vi "Main.vi"() -> ()   [LabVIEW 2018]
doc: "This Continuous Measurement sample project is based on the Queued Message Handler template.\n\nThe Event Handling Loop generates messages based on user interface actions.\n\nThe Message Handling Loop processes messages generated by the Event Handling Loop, or by other messages. There are also Acquisition and Logging message handling loop subVIs, and a chart updating loop."
uses:
  Controls/Acquired Data.ctl
  Controls/Time Remaining.ctl
  Controls/UI State.ctl
  Settings/Settings.ctl
  Acquisition/Hardware Configuration.ctl
  Logging/Logging Configuration.ctl
  <vilib>/addons/database/Connection.llb/Conn ObjectReference.ctl
  Support/Message Queue/Enqueue Message (Array).vi
  Support/Message Queue/Enqueue Message (Single).vi
  <vilib>/Utility/error.llb/Error Cluster From Error Code.vi
  <vilib>/ErrorRing/Error Ring.xnode
  Logging/Logging.lvlib
  Acquisition/Acquisition.lvlib
  Settings/Settings.lvlib
  support/User Event - Stop/User Event - Stop.lvlib
  support/Message Queue/Message Queue.lvlib
  <vilib>/addons/database/NI_Database_API.lvlib
  OSTEP_MySQLdBTools/MySQLTools.lvlib
  Settings/Settings Dialog.vi
panel:
  in  "UI State":T1
  out "Test In Progress":bool
  out "Time":T2 format="%<00:%M:%S>T"
  in  "Operator":u16(ring) items=["Select Operator"=0, "Wally Taylor"=2, "Max Ivanov"=3, "Scott Mowery"=4, "Robert Heitsenrether"=5, "Chris Haith"=6, "Chris McGrath"=7, "Kevin Harrison"=8, "Nathan Holcomb"=9, "Warren Krug"=10, "Winston Hensley"=11]
  in  "Location":u16(ring) items=["Chesapeake", "Silver Spring", "Gulf", "Seattle"]
  out "StatusBox":string
  out "Data":dbl(graph)
  in  "Range Data":T3={"offset"=99.0, "time"=""} {"offset" format="%.3g"}
  out "User Event - Stop":refnum<user-event>
  in  "Settings":bool
  in  "Start":bool
  in  "Stop":bool
  out "Status Bar":string
  in  "Exit":bool
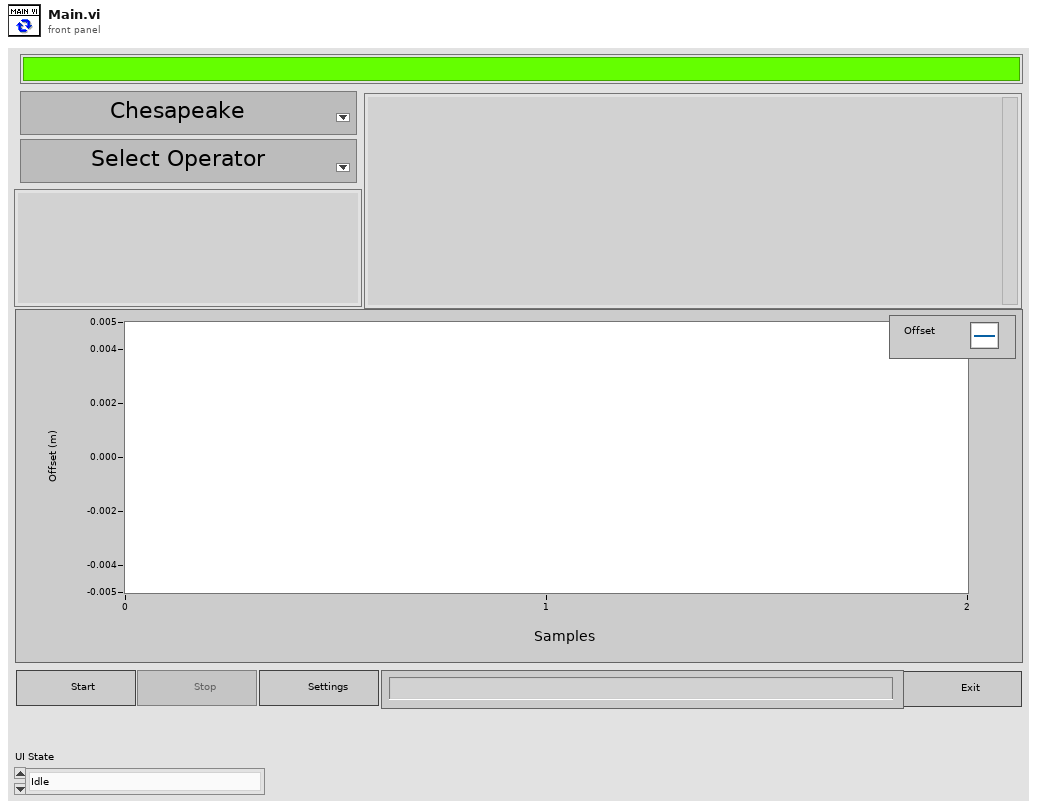
[diagram p1: front panel]
types:
  T1 = typedef "UI State.ctl" = enum16{"Idle", "Acquiring and Logging", "Waiting for Exit", "Waiting for Exit (Acq Stopped)", "Waiting for Exit (Log Stopped)", "Waiting for Stop", "Waiting for Stop (Acq Stopped)", "Waiting for Stop (Log Stopped)"}
  T2 = typedef "Time Remaining.ctl" = timestamp
  T3 = typedef "Acquired Data.ctl" = cluster{"offset":dbl, "time":string}
  T4 = typedef "Settings.lvlib/Settings.ctl" = cluster{"Hardware Configuration":T5, "Logging Configuration":T6, "UI Refs":cluster{"Start Ref":refnum<vi>, "Settings Ref":refnum<vi>, "Stop Ref":refnum<vi>, "Exit Ref":refnum<vi>, "Status Ref":refnum<vi>, "Data Ref":refnum<vi>, "StatusBox Ref":refnum<vi>, "Location Ref":refnum<vi>, "Operator Ref":refnum<vi>, "Time Ref":refnum<vi>, "Test in Progess Ref":refnum<vi>}, "Calibration Data":cluster{"calibrationID":u16, "operatorID":u16, "sensorID":u16, "start_time":string, "end_time":string, "offset":dbl, "offset_units":string, "ring_time":dbl, "error":dbl, "Passed":u8, "data_storage_location":string, "comments":string}, "Time Elapsed":u16, "Samples Required":u16}
  T5 = typedef "Acquisition.lvlib/Hardware Configuration.ctl" = cluster{"COM Port":refnum<visa-resource-name>, "Reference Distance":dbl, "Sensor SN":string}
  T6 = typedef "Logging.lvlib/Logging Configuration.ctl" = cluster{"Log File Base Path":path, "Datafile Ref":refnum<file>, "Database Ref":T7}
  T7 = typedef "NI_Database_API.lvlib/Conn ObjectReference.ctl" = refnum<k1>
  T8 = typedef "Message Queue.lvlib/All Message Queues.ctl" = cluster{"Message Queues":cluster{"UI":refnum<queue>, "Acquisition":refnum<queue>, "Logging":refnum<queue>}, "Data Queues & Notifier":cluster{"Data Queue":T9, "Data Notifer":T10}}
  T9 = typedef "Data Queue.ctl" = refnum<queue>
  T10 = typedef "Data Notifier.ctl" = refnum<notifier>
  T11 = typedef "MySQLTools.lvlib/BasicOperatorInfo.ctl" = cluster{"Full Name":string, "Email":string, "Phone Number":string, "Operator ID":string}
  T12 = typedef "Operator Ring.ctl" = u16
  T13 = typedef "MySQLTools.lvlib/Sensor Data.ctl" = cluster{"sensorID":u16, "sensorType":string, "model_number":string, "serial_number":string, "precision":dbl, "accuracy":dbl, "datasheet_website":string, "units":string}
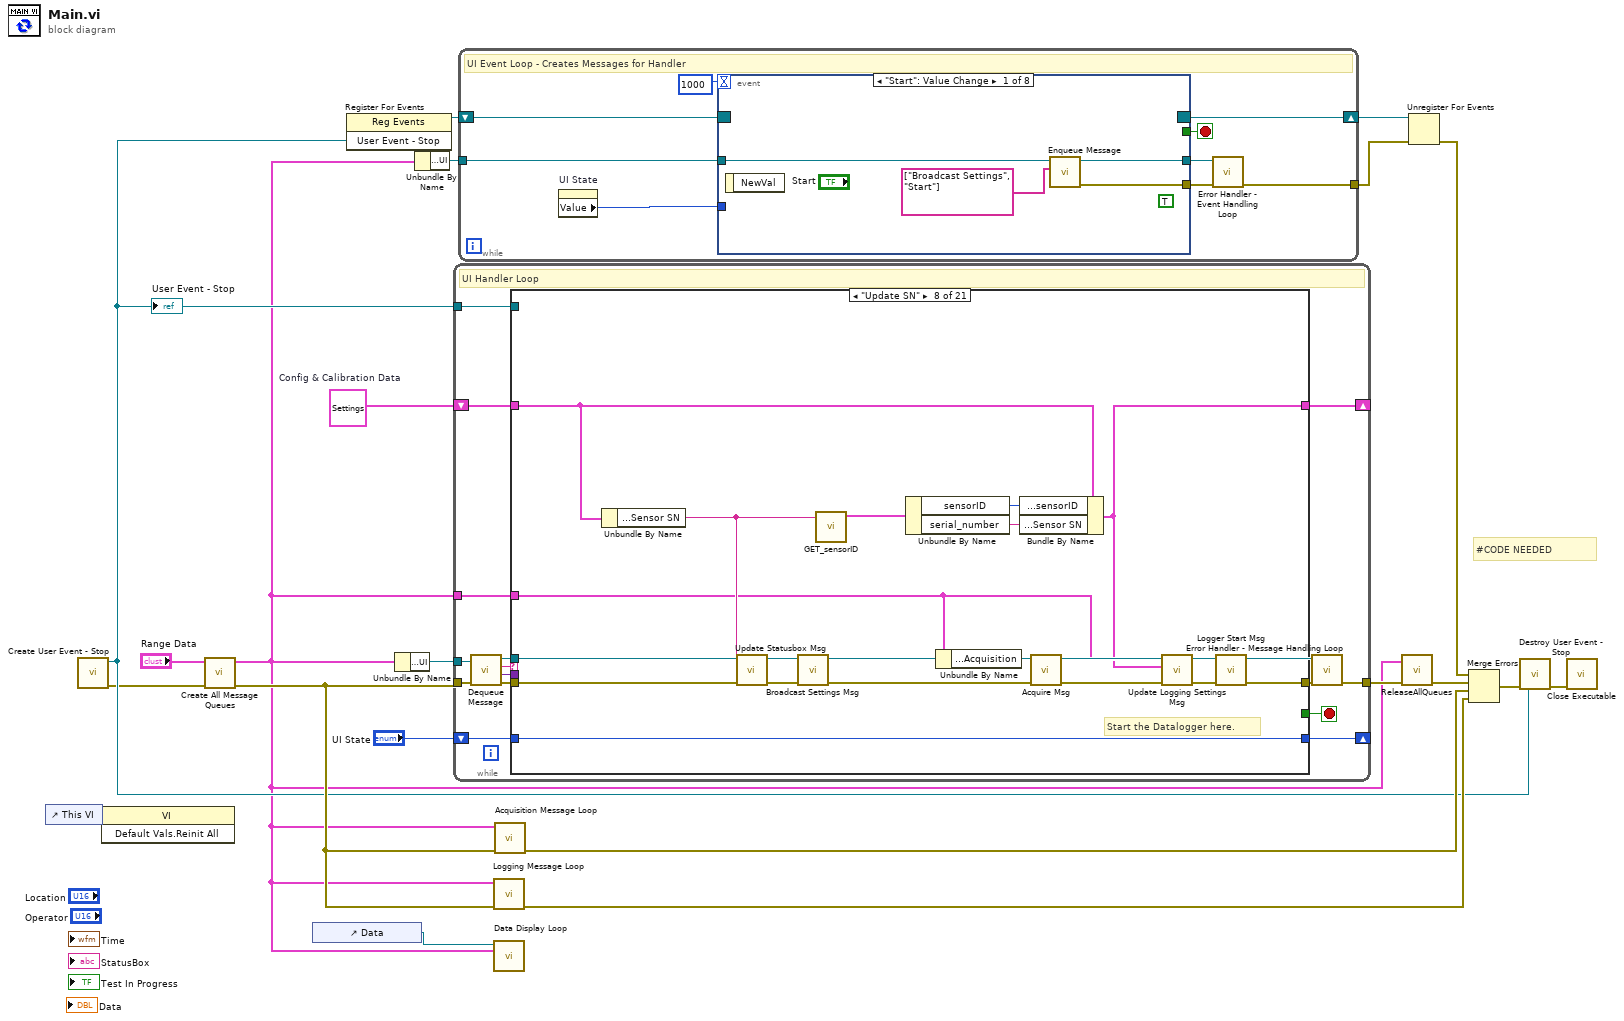
[diagram p0: block diagram]
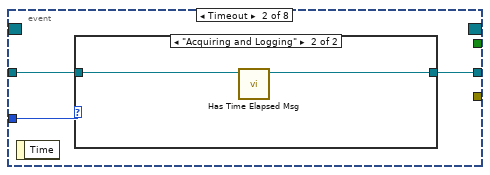
[diagram p2: hidden frame]
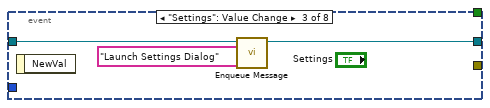
[diagram p4: hidden frame]
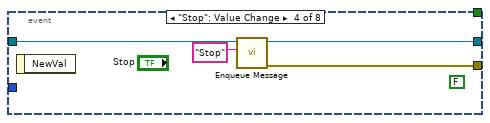
[diagram p5: hidden frame]
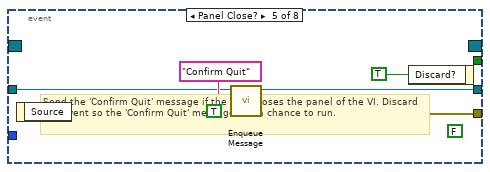
[diagram p6: hidden frame]
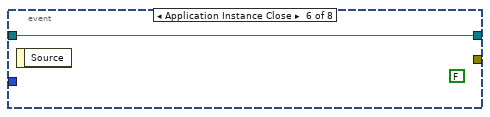
[diagram p7: hidden frame]
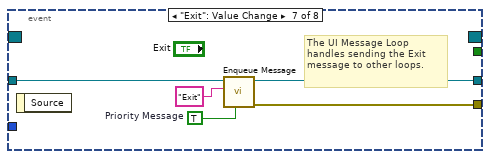
[diagram p8: hidden frame]
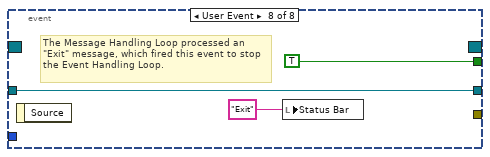
[diagram p9: hidden frame]
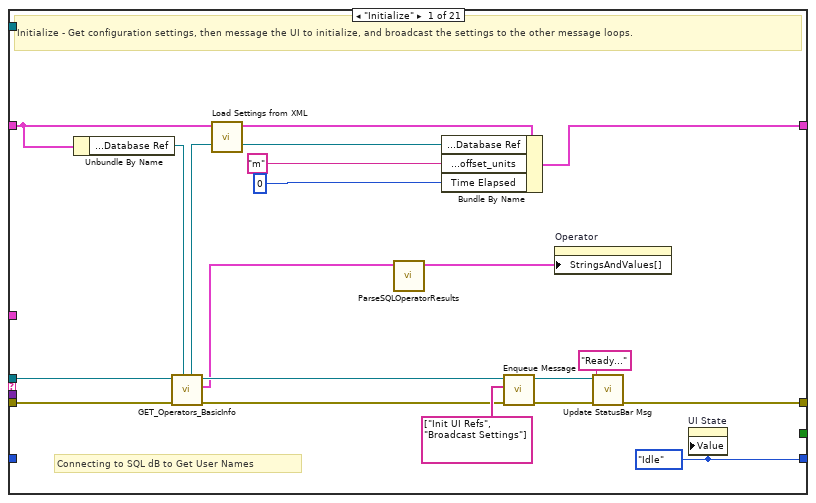
[diagram p10: hidden frame]
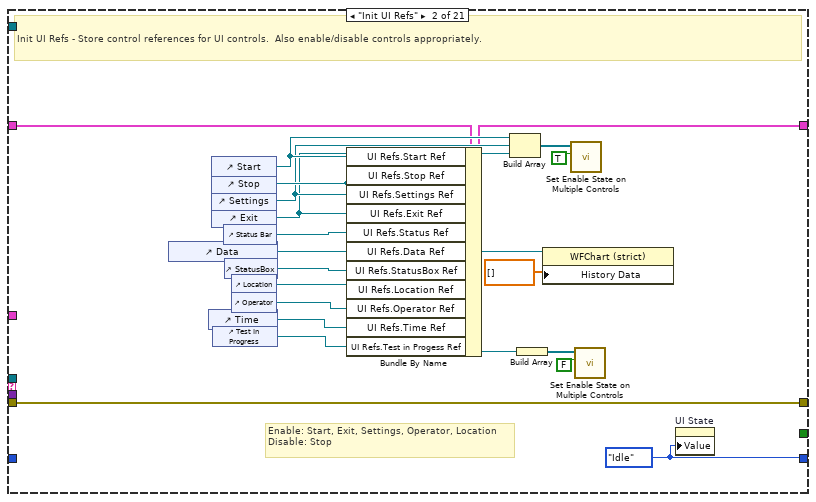
[diagram p11: hidden frame]
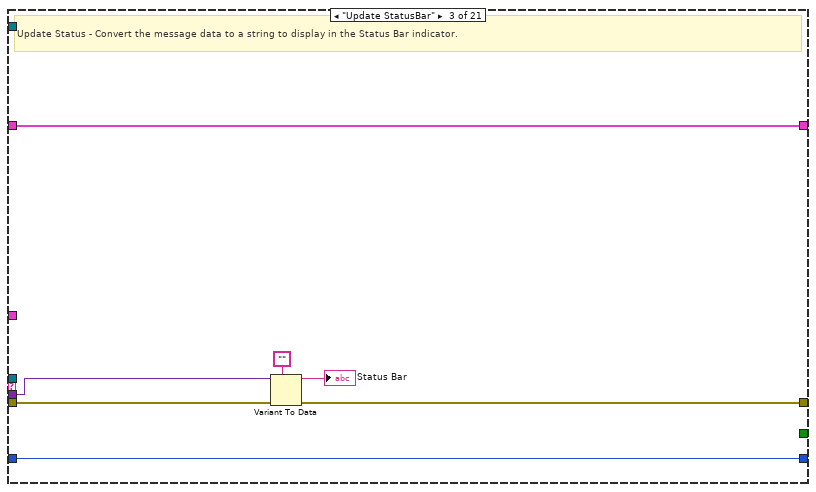
[diagram p12: hidden frame]
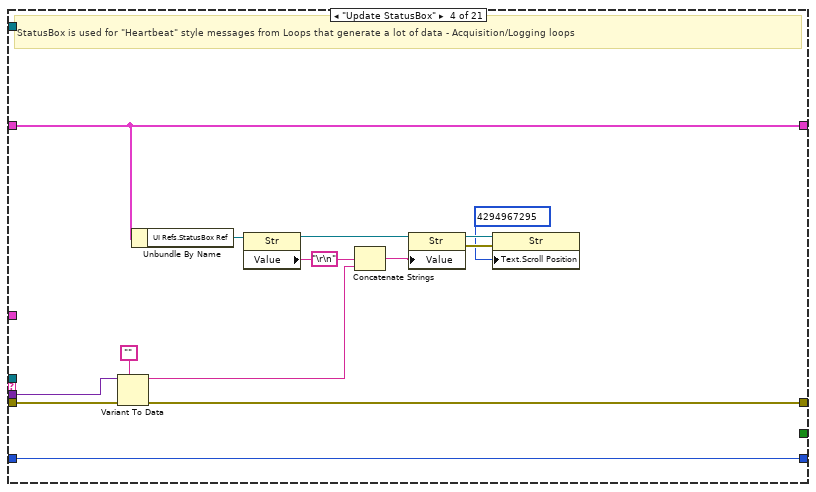
[diagram p13: hidden frame]
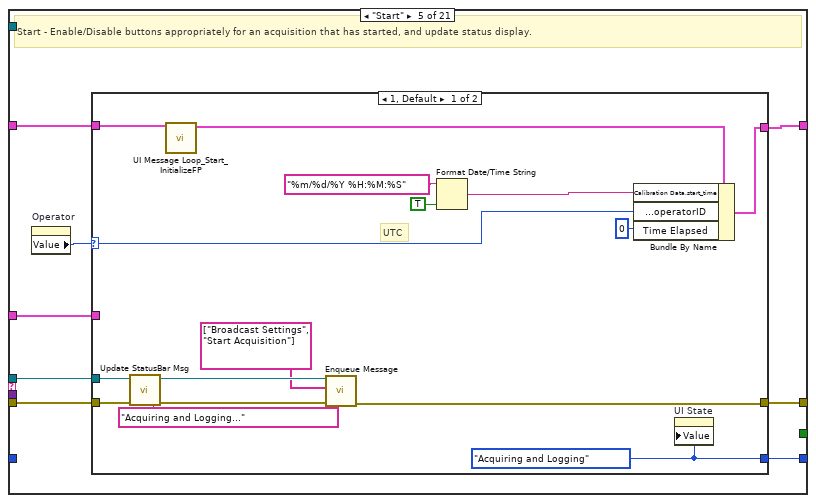
[diagram p14: hidden frame]
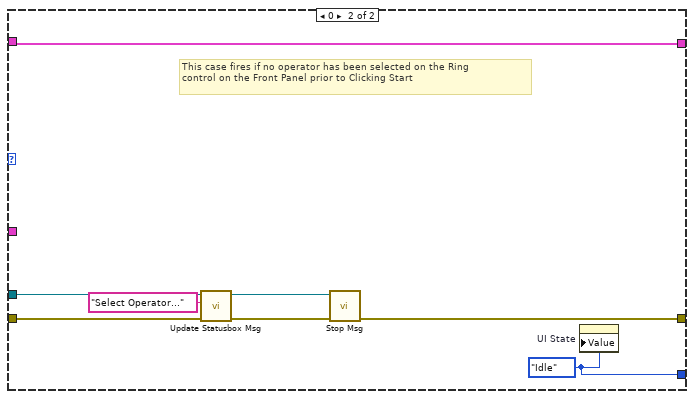
[diagram p15: hidden frame]
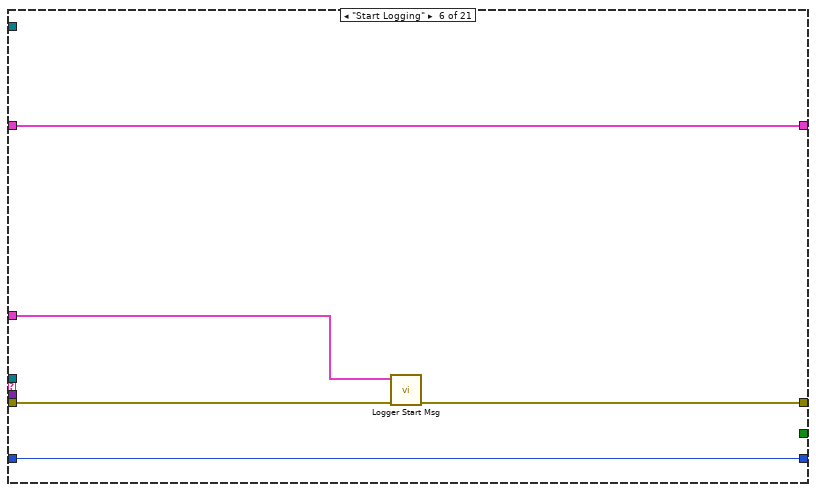
[diagram p16: hidden frame]
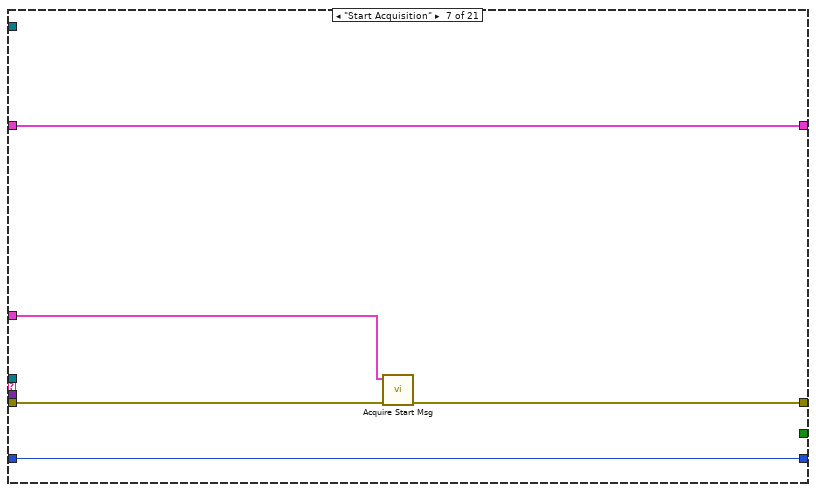
[diagram p17: hidden frame]
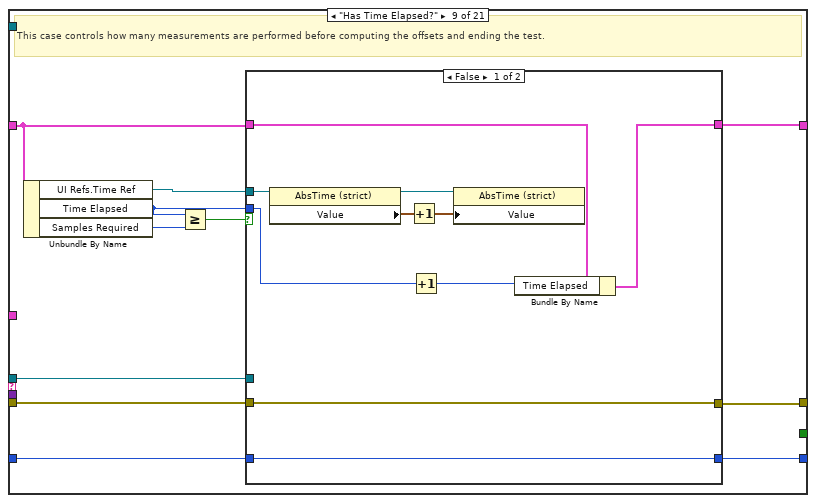
[diagram p18: hidden frame]
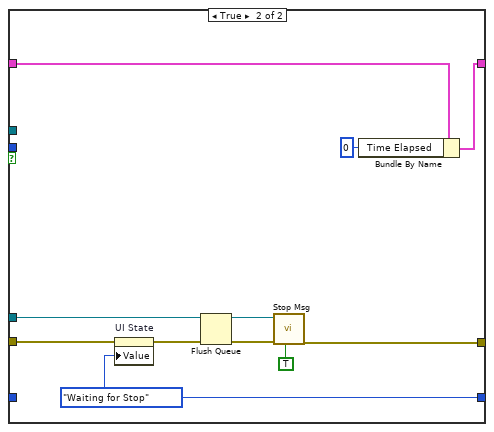
[diagram p19: hidden frame]
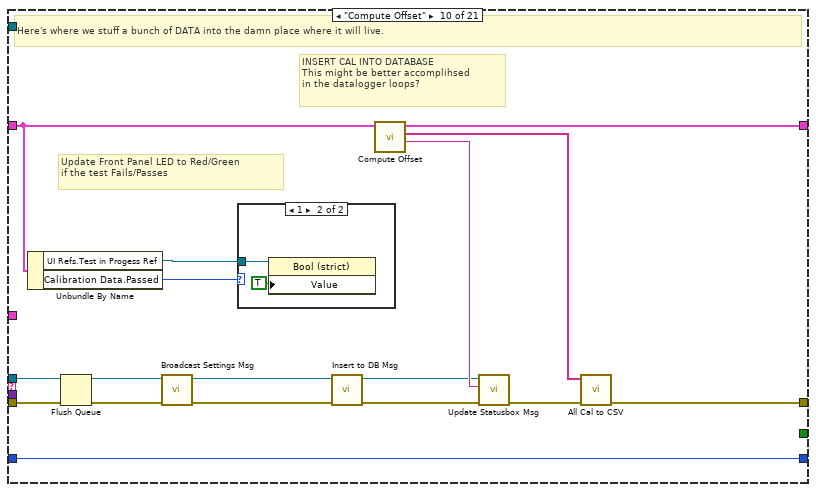
[diagram p20: hidden frame]
diagram:
  w1 = T4 {"Hardware Configuration"={"COM Port"="", "Reference Distance"=0.0, "Sensor SN"=""}, "Logging Configuration"={"Log File Base Path"=path "", "Datafile Ref"=refnum, "Database Ref"=refnum}, "UI Refs"={"Start Ref"=refnum, "Settings Ref"=refnum, "Stop Ref"=refnum, "Exit Ref"=refnum, "Status Ref"=refnum, "Data Ref"=refnum, "StatusBox Ref"=refnum, "Location Ref"=refnum, "Operator Ref"=refnum, "Time Ref"=refnum, "Test in Progess Ref"=refnum}, "Calibration Data"={"calibrationID"=0, "operatorID"=0, "sensorID"=0, "start_time"="", "end_time"="", "offset"=0.0, "offset_units"="", "ring_time"=0.0, "error"=0.0, "Passed"=0, "data_storage_location"="", "comments"=""}, "Time Elapsed"=0, "Samples Required"=480}  # Config & Calibration Data
  # "#CODE NEEDED"
  n1 = control-ref of="This VI"() -> (w6:refnum<vi>)
  n2 = call "Create User Event - Stop.vi"() -> ("error out"=w4:errorcluster, "User Event - Stop"=w8:refnum<user-event>)  [unwired: 10 in]
  "User Event - Stop" <- w8
  n3 = invoke class="VI" method="Default Vals.Reinit All"(reference=w6) -> ()  [unwired: 2 in, 3 out]
  n4 = call "Create All Message Queues.vi"("error in (no error)"=w4, "Data"="Range Data") -> ("error out"=w17:errorcluster, "Message Queues out"=w2:T8)  [unwired: 8 in]
  n5 = control-ref of="Data"() -> (w5:refnum<vi>)
  n6 = register-events(w8) -> (reference out=w9:refnum<event-registration>)  [unwired: 2 in, 1 out]
  n7 = Unbundle By Name(w2) -> ("Message Queues.UI"=w3:refnum<queue>)
  n8 = Unbundle By Name(w2) -> ("Message Queues.UI"=w12:refnum<queue>)
  n9 = while {
    tunnel: w8 -> [w35]
    shift-right: [w30] -> _
    shift-left: w1 -> [w29]
    shift-right: [w25] -> _
    shift-left: "UI State" -> [w26]
    tunnel: w17 -> [w34]
    tunnel: [w28] -> w21
    tunnel: w2 -> [w24]
    tunnel: w3 -> [w23]
    stop <- w36 stop-if-true
    # "UI Handler Loop"
    n10 = call "Dequeue Message.vi"("error in (no error)"=w34, "Message Queue"=w23) -> ("error out"=w33:errorcluster, "Message Data"=w31:variant, "Message"=w32:string, "dup Message Queue"=w22:refnum<queue>)  [unwired: 6 in]
    n11 = case "Message Cases" shown="\"Update SN\"" w32 {
      selector: w32 -> [_ _ _ _ _ _ _ _ _ _ _ _ _ _ _ _ _ _ _ _ w368]
      tunnel: w22 -> [w54 _ _ _ w100 _ _ w154 w167 w200 _ w224 w248 w269 w291 _ w308 _ w327 _ _]
      tunnel: w33 -> [w48 w56 w81 w85 w101 w130 w136 w155 w162 w199 w211 w227 w249 w270 w294 w299 w310 w316 w326 w358 _]
      tunnel: [w49 w56 w78 w84 w104 w129 w135 w150 w161 w202 w210 w243 w247 w268 w288 w302 w304 w319 w325 w364 w367] -> w27
      tunnel: [_ _ _ _ _ _ _ _ _ _ _ _ _ _ _ _ _ _ _ TRUE _] -> w36
      tunnel: w31 -> [_ _ w80 w82 _ _ _ _ _ _ _ _ _ _ w295 _ _ w320 _ w356 _]
      tunnel: w35 -> [_ _ _ _ _ _ _ _ _ _ _ _ _ _ _ _ _ _ _ w365 _]
      tunnel: [w37 w65 w77 w83 w98 w133 w138 w142 w165 w201 w217 w223 w251 w272 w292 w300 w307 w323 w329 w363 w370] -> w30
      tunnel: w29 -> [w39 w66 w77 w83 w99 w133 w138 w147 w166 w190 w217 w218 w251 w272 w293 w300 w311 w323 w329 w363 w370]
      tunnel: w26 -> [_ _ w76 w96 _ w132 w137 w156 w163 w205 w216 w234 w250 w271 w296 w301 w305 w318 w328 _ w369]
      tunnel: [w43 w55 w76 w96 w103 w132 w137 w156 w164 w205 w216 w228 w246 w267 w296 w301 w305 w318 w324 w350 w369] -> w25
      tunnel: w24 -> [_ _ _ _ w102 w131 w134 w143 _ _ w213 w233 _ _ _ w298 _ _ _ w354 _]
      frame "Initialize" {
        w43 = UI_State."Idle" ("UI State")
        # "Connecting to SQL dB to Get User Names"
        # "Initialize - Get configuration settings, then message the UI to initialize, and broadcast the settings to the other message loops."
        n12 = Unbundle By Name(w39) -> ("Logging Configuration.Database Ref"=w45:T7)
        n13 = call "GET_Operators_BasicInfo.vi"("Database Ref In"=w45, "error in (no error)"=w48) -> ("error out"=w47:errorcluster, "Basic Info"=w46:T11[], "Database Ref Out"=w44:T7)  [unwired: 7 in]
        n14 = call "Load Settings from XML.vi"("Settings in"=w39) -> ("Settings out"=w38:T4)  [unwired: 9 in, 1 out]
        n15 = call "ParseSQLOperatorResults.vi"("Basic Info"=w46) -> ("Array"=w41:cluster{"Full Name":string, "Numeric":i32}[])  [unwired: 10 in]
        n16 = Bundle By Name(cluster=w38, "Logging Configuration.Database Ref"=w44, "Calibration Data.offset_units"="m", "Time Elapsed"=u16 0) -> (w37:T4)
        n17 = call-poly "Enqueue Message.vi"("error in (no error)"=w47, "Message Array"=string[] ["Init UI Refs", "Broadcast Settings"], "Message Queue"=w54) -> ("error out"=w50:errorcluster, "dup Message Queue"=w52:refnum<queue>)  [unwired: 7 in]
        n18 = property on="Operator" class="Ring (strict)"("StringsAndValues[]"=w41) -> ()  [unwired: 2 in, 2 out]
        n19 = call "Update StatusBar Msg.vi"("error in (no error)"=w50, "Ready..."="Ready...", "Queue in"=w52) -> ("error out"=w49:errorcluster)  [unwired: 7 in, 1 out]
        n20 = property on="UI State" class="Enum (strict)"("Value"=w43) -> ()  [unwired: 2 in, 2 out]
      }
      frame "Init UI Refs" {
        w55 = UI_State."Idle" ("UI State")
        # "Enable: Start, Exit, Settings, Operator, Location\nDisable: Stop"
        # "Init UI Refs - Store control references for UI controls.  Also enable/disable controls appropriately."
        n21 = control-ref of="Data"() -> (w58:refnum<vi>)
        n22 = control-ref of="Time"() -> (w63:refnum<vi>)
        n23 = control-ref of="Start"() -> (w69:refnum<vi>)
        n24 = control-ref of="Stop"() -> (w70:refnum<vi>)
        n25 = control-ref of="Settings"() -> (w68:refnum<vi>)
        n26 = control-ref of="Exit"() -> (w67:refnum<vi>)
        n27 = control-ref of="Test In Progress"() -> (w64:refnum<vi>)
        n28 = control-ref of="Status Bar"() -> (w59:refnum<vi>)
        n29 = control-ref of="StatusBox"() -> (w60:refnum<vi>)
        n30 = control-ref of="Location"() -> (w61:refnum<vi>)
        n31 = control-ref of="Operator"() -> (w62:refnum<vi>)
        n32 = Bundle By Name(cluster=w66, "UI Refs.Start Ref"=w69, "UI Refs.Stop Ref"=w70, "UI Refs.Settings Ref"=w68, "UI Refs.Exit Ref"=w67, "UI Refs.Status Ref"=w59, "UI Refs.Data Ref"=w58, "UI Refs.StatusBox Ref"=w60, "UI Refs.Location Ref"=w61, "UI Refs.Operator Ref"=w62, "UI Refs.Time Ref"=w63, "UI Refs.Test in Progess Ref"=w64) -> (w65:T4)
        n33 = Build Array(w69, w68, w67) -> (w73:refnum<vi>[])
        n34 = Build Array(w70) -> (w72:refnum<vi>[])
        n35 = property class="WFChart (strict)"(reference=w58, "History Data"=dbl[] []) -> ()  [unwired: 1 in, 2 out]
        n36 = call "Set Enable State on Multiple Controls.vi"("Enable?"=TRUE, "Controls"=w73) -> ()  [unwired: 10 in]
        n37 = call "Set Enable State on Multiple Controls.vi"("Enable?"=FALSE, "Controls"=w72) -> ()  [unwired: 10 in]
        n38 = property on="UI State" class="Enum (strict)"("Value"=w55) -> ()  [unwired: 2 in, 2 out]
      }
      frame "Update StatusBar" {
        # "Update Status - Convert the message data to a string to display in the Status Bar indicator."
        n39 = Variant To Data(error in=w81, type="", Variant=w80) -> (data=→"Status Bar":string, error out=w78:errorcluster)
      }
      frame "Update StatusBox" {
        # "StatusBox is used for \"Heartbeat\" style messages from Loops that generate a lot of data - Acquisition/Logging loops"
        n40 = Variant To Data(error in=w85, type="", Variant=w82) -> (data=w90:string, error out=w84:errorcluster)
        n41 = Unbundle By Name(w83) -> ("UI Refs.StatusBox Ref"=w86:refnum<vi>)
        n42 = property class="Str"(reference=w86) -> (reference out=w94:refnum<vi>, "Value"=w93:string)  [unwired: 1 in, 1 out]
        n43 = Concatenate Strings(w93, "\r\n", w90) -> (w91:string)
        n44 = property class="Str"(reference=w94, "Value"=w91) -> (reference out=w89:refnum<vi>, error out=w88:errorcluster)  [unwired: 1 in]
        n45 = property class="Str"(reference=w89, error in=w88, "Text.Scroll Position"=u32 4294967295) -> ()  [unwired: 2 out]
      }
      frame "Start" {
        # "Start - Enable/Disable buttons appropriately for an acquisition that has started, and update status display."
        n46 = property on="Operator" class="Ring (strict)"() -> ("Value"=w97:T12)  [unwired: 2 in, 2 out]
        n47 = case shown="1, Default" w97 {
          selector: w97 -> [w108 _]
          tunnel: [w107 w125] -> w104
          tunnel: [w116 w121] -> w103
          tunnel: w102 -> [_ _]
          tunnel: w101 -> [w120 w128]
          tunnel: w99 -> [w117 w122]
          tunnel: w100 -> [w118 w123]
          tunnel: [w113 w122] -> w98
          frame 1, Default {
            w116 = UI_State."Acquiring and Logging" ("UI State")
            # "UTC"
            n48 = call "Update StatusBar Msg.vi"("error in (no error)"=w120, "Ready..."="Acquiring and Logging..." ("Acquiring and Logging..."), "Queue in"=w118) -> ("error out"=w109:errorcluster, "Queue out"=w110:refnum<queue>)  [unwired: 7 in]
            n49 = call "UI Message Loop_Start_InitializeFP.vi"("C&C Data in"=w117) -> ("C&C Data out"=w111:T4)  [unwired: 10 in]
            n50 = call-poly "Enqueue Message.vi"("error in (no error)"=w109, "Message Array"=string[] ["Broadcast Settings", "Start Acquisition"], "Message Queue"=w110) -> ("error out"=w107:errorcluster)  [unwired: 7 in, 1 out]
            n51 = Format Date/Time String(time format string (%c)="%m/%d/%Y %H:%M:%S" ("string"), UTC format=TRUE) -> (date/time string=w112:string)  [unwired: 1 in]
            n52 = Bundle By Name(cluster=w111, "Calibration Data.start_time"=w112, "Calibration Data.operatorID"=w108, "Time Elapsed"=u16 0) -> (w113:T4)
            n53 = property on="UI State" class="Enum (strict)"("Value"=w116) -> ()  [unwired: 2 in, 2 out]
          }
          frame 0 {
            w121 = UI_State."Idle" ("UI State")
            # "This case fires if no operator has been selected on the Ring\ncontrol on the Front Panel prior to Clicking Start"
            n54 = call "Update Statusbox Msg.vi"("error in (no error)"=w128, "Message"="Select Operator...", "Queue in"=w123) -> ("error out"=w126:errorcluster, "Queue out"=w127:refnum<queue>)  [unwired: 7 in]
            n55 = call "Stop Msg.vi"("error in (no error)"=w126, "Queue in"=w127) -> ("error out"=w125:errorcluster)  [unwired: 8 in, 1 out]
            n56 = property on="UI State" class="Enum (strict)"("Value"=w121) -> ()  [unwired: 2 in, 2 out]
          }
        }
      }
      frame "Start Logging" {
        n57 = call "Logger Start Msg.vi"("error in (no error)"=w130, "Message Queues in"=w131) -> ("error out"=w129:errorcluster)  [unwired: 8 in, 1 out]
      }
      frame "Start Acquisition" {
        n58 = call "Acquire Start Msg.vi"("error in (no error)"=w136, "Message Queues in"=w134) -> ("error out"=w135:errorcluster)  [unwired: 8 in, 1 out]
      }
      frame "Update SN" {
        # "Start the Datalogger here."
        n59 = Unbundle By Name(w147) -> ("Hardware Configuration.Sensor SN"=w146:string)
        n60 = call "Update Statusbox Msg.vi"("error in (no error)"=w155, "Message"=w146, "Queue in"=w154) -> ("error out"=w144:errorcluster, "Queue out"=w149:refnum<queue>)  [unwired: 7 in]
        n61 = call "Broadcast Settings Msg.vi"("error in (no error)"=w144, "Queue in"=w149) -> ("error out"=w148:errorcluster)  [unwired: 8 in, 1 out]
        n62 = call "GET_sensorID.vi"("Serial Number"=w146) -> ("Sensor Data out"=w152:T13)  [unwired: 9 in, 1 out]
        n63 = Unbundle By Name(w152) -> ("sensorID"=w151:u16, "serial_number"=w145:string)
        n64 = Unbundle By Name(w143) -> ("Message Queues.Acquisition"=w153:refnum<queue>)
        n65 = Bundle By Name(cluster=w147, "Calibration Data.sensorID"=w151, "Hardware Configuration.Sensor SN"=w145) -> (w142:T4)
        n66 = call "Acquire Msg.vi"("error in (no error)"=w148, "Queue in"=w153) -> ("error out"=w141:errorcluster)  [unwired: 9 in]
        n67 = call "Update Logging Settings Msg.vi"("error in (no error)"=w141, "Config"=w142, "Message Queues in"=w143) -> ("error out"=w140:errorcluster, "Message Queues out"=w139:T8)  [unwired: 7 in]
        n68 = call "Logger Start Msg.vi"("error in (no error)"=w140, "Message Queues in"=w139) -> ("error out"=w150:errorcluster)  [unwired: 8 in, 1 out]
      }
      frame "Has Time Elapsed?" {
        # "This case controls how many measurements are performed before computing the offsets and ending the test."
        n69 = Unbundle By Name(w166) -> ("UI Refs.Time Ref"=w160:refnum<vi>, "Time Elapsed"=w157:u16, "Samples Required"=w159:u16)
        n70 = Greater Or Equal?(x=w157, y=w159) -> (x >= y?=w158:bool)
        n71 = case "Has Time Elapsed Yet?" shown="False" w158 {
          tunnel: w167 -> [_ w186]
          tunnel: w166 -> [w175 w188]
          tunnel: [w174 w187] -> w165
          tunnel: [w177 w181] -> w164
          tunnel: w163 -> [w177 _]
          tunnel: w162 -> [w176 w179]
          tunnel: [w176 w178] -> w161
          tunnel: w160 -> [w172 _]
          tunnel: w157 -> [w168 _]
          frame False {
            n72 = property class="AbsTime (strict)"(reference=w172) -> (reference out=w171:refnum<vi>, "Value"=w170:T2)  [unwired: 1 in, 1 out]
            n73 = Increment(x=w170) -> (x+1=w169:T2)
            n74 = Increment(x=w168) -> (x+1=w173:u16)
            n75 = property class="AbsTime (strict)"(reference=w171, "Value"=w169) -> ()  [unwired: 1 in, 2 out]
            n76 = Bundle By Name(cluster=w175, "Time Elapsed"=w173) -> (w174:T4)
          }
          frame True {
            w181 = UI_State."Waiting for Stop" ("UI State")
            # "Reset the Timer"
            n77 = property on="UI State" class="Enum (strict)"(error in=w179, "Value"=w181) -> (error out=w180:errorcluster)  [unwired: 1 in, 1 out]
            n78 = Flush Queue(queue=w186, error in (no error)=w180) -> (queue out=w184:refnum<queue>, error out=w185:errorcluster)  [unwired: 1 out]
            n79 = call "Stop Msg.vi"("Priority Message? (F)"=TRUE, "error in (no error)"=w185, "Queue in"=w184) -> ("error out"=w178:errorcluster)  [unwired: 7 in, 1 out]
            n80 = Bundle By Name(cluster=w188, "Time Elapsed"=u16 0) -> (w187:T4)
          }
        }
      }
      frame "Compute Offset" {
        # "Update Front Panel LED to Red/Green\nif the test Fails/Passes"
        # "INSERT CAL INTO DATABASE\nThis might be better accomplihsed\nin the datalogger loops?"
        # "Here's where we stuff a bunch of DATA into the damn place where it will live."
        n81 = Unbundle By Name(w190) -> ("UI Refs.Test in Progess Ref"=w189:refnum<vi>, "Calibration Data.Passed"=w191:u8)
        n82 = Flush Queue(queue=w200, error in (no error)=w199) -> (queue out=w196:refnum<queue>, error out=w195:errorcluster)  [unwired: 1 out]
        n83 = call "Broadcast Settings Msg.vi"("error in (no error)"=w195, "Queue in"=w196) -> ("error out"=w198:errorcluster, "Queue out"=w197:refnum<queue>)  [unwired: 8 in]
        n84 = case shown="1" w191 {
          tunnel: w189 -> [w207 w208]
          frame 0, Default {
            n85 = property class="Bool (strict)"(reference=w207, "Value"=FALSE) -> ()  [unwired: 1 in, 2 out]
          }
          frame 1 {
            n86 = property class="Bool (strict)"(reference=w208, "Value"=TRUE) -> ()  [unwired: 1 in, 2 out]
          }
        }
        n87 = call "Insert to DB Msg.vi"("error in (no error)"=w198, "UI Queue in"=w197) -> ("error out"=w193:errorcluster, "UI Queue out"=w194:refnum<queue>)  [unwired: 8 in]
        n88 = call "Compute Offset.vi"("C&C Data in"=w190) -> ("Test Results"=w204:string, "Test Result Array"=w203:string[], "C&C Data out"=w201:T4)  [unwired: 8 in]
        n89 = call "Update Statusbox Msg.vi"("error in (no error)"=w193, "Message"=w204, "Queue in"=w194) -> ("error out"=w192:errorcluster)  [unwired: 7 in, 1 out]
        n90 = call "All Cal to CSV.vi"("error in (no error)"=w192, "Array"=w203) -> ("error out"=w202:errorcluster)  [unwired: 9 in]
      }
      frame "Insert Calibration to dB" {
        # "Make sure you update settings in Logging Loop prior to calling this case."
        n91 = Unbundle By Name(w213) -> ("Message Queues.Logging"=w212:refnum<queue>)
        n92 = call-poly "Enqueue Message.vi"("Priority Message? (F)"=TRUE, "error in (no error)"=w211, "Message"="Insert Cal", "Message Queue"=w212) -> ("error out"=w210:errorcluster)  [unwired: 6 in, 1 out]
      }
      frame "Stop" {
        # "Stop - Enable/Disable buttons appropriately for an acquisition that has stopped, and update status"
        n93 = Unbundle By Name(w233) -> ("Message Queues.Logging"=w229:refnum<queue>, "Message Queues.Acquisition"=w232:refnum<queue>)
        n94 = Unbundle By Name(w218) -> ("UI Refs.Stop Ref"=w238:refnum<vi>, "UI Refs.Start Ref"=w237:refnum<vi>, "UI Refs.Exit Ref"=w236:refnum<vi>, "UI Refs.Settings Ref"=w235:refnum<vi>)
        n95 = call "Stop Msg.vi"("Priority Message? (F)"=TRUE, "error in (no error)"=w227, "Queue in"=w232) -> ("error out"=w230:errorcluster)  [unwired: 8 in]
        n96 = Build Array(w237, w236, w235) -> (w241:refnum<vi>[])
        n97 = Build Array(w238) -> (w240:refnum<vi>[])
        n98 = call "Set Enable State on Multiple Controls.vi"("Enable?"=FALSE, "Controls"=w240) -> ()  [unwired: 10 in]
        n99 = call "Set Enable State on Multiple Controls.vi"("Enable?"=TRUE, "Controls"=w241) -> ()  [unwired: 10 in]
        n100 = call "Stop Msg.vi"("error in (no error)"=w230, "Queue in"=w229) -> ("error out"=w226:errorcluster)  [unwired: 9 in]
        n101 = case shown="Default" w234 {
          selector: w234 -> [w244 _]
          tunnel: [w244 UI_State."Idle" ("UI State")] -> w228
          frame "Waiting for Exit" {
          }
          frame Default {
          }
        }
        n102 = call-poly "Enqueue Message.vi"("error in (no error)"=w226, "Message Array"=string[] ["Broadcast Settings", "Compute Offset"], "Message Queue"=w224) -> ("error out"=w225:errorcluster)  [unwired: 7 in, 1 out]
        n103 = Format Date/Time String(time format string (%c)="%m/%d/%Y %H:%M:%S" ("string"), UTC format=TRUE) -> (date/time string=w220:string)  [unwired: 1 in]
        n104 = Bundle By Name(cluster=w218, "Calibration Data.end_time"=w220) -> (w223:T4)
        n105 = Merge Errors(w225) -> (w243:errorcluster)
        n106 = property on="UI State" class="Enum (strict)"("Value"=w228) -> ()  [unwired: 2 in, 2 out]
      }
      frame "Acquisition Stopped" {
        # "Logic for determining what action to take when the acquisition has stopped."
        n107 = case shown="\"Waiting for Stop\", \"Waiting for Stop (Acq Stopped)\"" w250 {
          selector: w250 -> [w253 _ _ _ _]
          tunnel: w249 -> [w252 w255 w257 w260 w264]
          tunnel: w248 -> [_ _ _ w259 w265]
          tunnel: [w253 UI_State."Waiting for Exit (Acq Stopped)" ("UI State") UI_State."Waiting for Stop (Acq Stopped)" ("UI State") UI_State."Idle" ("UI State") UI_State."Idle" ("UI State")] -> w246
          tunnel: [w252 w255 w257 w258 w263] -> w247
          frame Default {
          }
          frame "Waiting for Exit", "Waiting for Exit (Acq Stopped)" {
          }
          frame "Waiting for Stop", "Waiting for Stop (Acq Stopped)" {
          }
          frame "Waiting for Exit (Log Stopped)" {
            # "If we are waiting to exit, and the logging has already stopped, then the \"Acquisition Stopped\" message indicates that it is time to exit."
            n108 = call "Exit Msg.vi"("error in (no error)"=w260, "Queue in"=w259) -> ("error out"=w258:errorcluster)  [unwired: 9 in]
          }
          frame "Waiting for Stop (Log Stopped)" {
            # "If we are waiting to stop, and the logging has already stopped, then the \"Acquisition Stopped\" message indicates that it is time to stop."
            n109 = call "Update StatusBar Msg.vi"("error in (no error)"=w264, "Ready..."="Ready...", "Queue in"=w265) -> ("error out"=w263:errorcluster)  [unwired: 7 in, 1 out]
          }
        }
        n110 = property on="UI State" class="Enum (strict)"("Value"=w246) -> ()  [unwired: 2 in, 2 out]
      }
      frame "Logging Stopped" {
        # "Logic for determining what action to take when the logging has stopped."
        n111 = case shown="\"Waiting for Exit (Acq Stopped)\"" w271 {
          selector: w271 -> [w274 _ _ _ _]
          tunnel: w270 -> [w273 w276 w278 w282 w285]
          tunnel: w269 -> [_ _ _ w280 w284]
          tunnel: [w274 UI_State."Waiting for Exit (Log Stopped)" ("UI State") UI_State."Waiting for Stop (Log Stopped)" ("UI State") UI_State."Idle" ("UI State") UI_State."Idle" ("UI State")] -> w267
          tunnel: [w273 w276 w278 w281 w283] -> w268
          frame Default {
          }
          frame "Waiting for Exit", "Waiting for Exit (Log Stopped)" {
          }
          frame "Waiting for Stop", "Waiting for Stop (Log Stopped)" {
          }
          frame "Waiting for Exit (Acq Stopped)" {
            n112 = call "Exit Msg.vi"("error in (no error)"=w282, "Queue in"=w280) -> ("error out"=w281:errorcluster)  [unwired: 9 in]
          }
          frame "Waiting for Stop (Acq Stopped)" {
            n113 = call "Update StatusBar Msg.vi"("error in (no error)"=w285, "Ready..."="Ready...", "Queue in"=w284) -> ("error out"=w283:errorcluster)  [unwired: 7 in, 1 out]
          }
        }
        n114 = property on="UI State" class="Enum (strict)"("Value"=w267) -> ()  [unwired: 2 in, 2 out]
      }
      frame "Update Config" {
        n115 = Variant To Data(error in=w294, type=w293, Variant=w295) -> (data=w292:T4, error out=w289:errorcluster)
        n116 = call-poly "Enqueue Message.vi"("error in (no error)"=w289, "Message"="Broadcast Settings", "Message Queue"=w291) -> ("error out"=w288:errorcluster)  [unwired: 7 in, 1 out]
      }
      frame "Broadcast settings" {
        # "Broadcast settings - Send the 'Update Settings' message to the Logging and Acquisition message loops."
        n117 = call "Update Acquisition Settings Msg.vi"("error in (no error)"=w299, "Config"=w300, "Message Queues in"=w298) -> ("error out"=w303:errorcluster, "Message Queues out"=w297:T8)  [unwired: 7 in]
        n118 = call "Update Logging Settings Msg.vi"("error in (no error)"=w303, "Config"=w300, "Message Queues in"=w297) -> ("error out"=w302:errorcluster)  [unwired: 7 in, 1 out]
      }
      frame "Launch Settings Dialog" {
        # "Launch Settings Dialog - Launch the Settings Dialog when the user clicks the 'Settings' button."
        n119 = call-by-ref "?"("error in (no error)"=w310, "Settings in"=w311) -> ("error out"=w306:errorcluster, "Cancelled?"=w309:bool, "Settings out"=w307:T4)  [unwired: 8 in, 3 out]
        n120 = case shown="False" w309 {
          tunnel: w308 -> [w314 _]
          tunnel: w306 -> [w313 w315]
          tunnel: [w312 w315] -> w304
          frame False {
            n121 = call "Broadcast Settings Msg.vi"("error in (no error)"=w313, "Queue in"=w314) -> ("error out"=w312:errorcluster)  [unwired: 8 in, 1 out]
          }
          frame True {
          }
        }
      }
      frame "Error" {
        # "Error - Display an error dialog. This message is sent by the \"Error Handler\" VIs at the end of other loops in this application."
        n122 = Variant To Data(error in=w316, type=errorcluster {"status"=FALSE, "code"=0, "source"=""} ("error constant"), Variant=w320) -> (data=w317:errorcluster, error out=w321:errorcluster)
        n123 = call <vilib>:"Simple Error Handler.vi"("error in (no error)"=w317) -> ()  [unwired: 4 in, 5 out]
        n124 = Merge Errors(w321) -> (w319:errorcluster)
      }
      frame "Confirm Quit" {
        # "Confirm Quit - Message that can confirm whether or not the user wants to exit the application."
        n125 = case shown="\"Acquiring and Logging\"" w328 {
          tunnel: w327 -> [w335 w339]
          tunnel: w326 -> [w334 w338]
          tunnel: [w333 w337] -> w325
          tunnel: [UI_State."Idle" ("UI State") w336] -> w324
          frame Default {
            # "If 'Confirm Quit' comes in while the system is idle, there is no need for a confirmation message."
            n126 = call-poly "Enqueue Message.vi"("Priority Message? (F)"=TRUE, "error in (no error)"=w334, "Message"="Exit", "Message Queue"=w335) -> ("error out"=w333:errorcluster)  [unwired: 6 in, 1 out]
          }
          frame "Acquiring and Logging" {
            n127 = Two Button Dialog(message="Are you sure you want to quit while the acquisition is running?" ("Confirm Quit Message"), 1:"No" ("No"), 2:"Yes" ("Yes")) -> (T button?=w340:bool)
            n128 = case shown="True" w340 {
              tunnel: w339 -> [_ w348]
              tunnel: w338 -> [w345 w349]
              tunnel: [w345 w347] -> w337
              tunnel: [UI_State."Acquiring and Logging" ("UI State") UI_State."Waiting for Exit" ("UI State")] -> w336
              frame False {
                # "User did not want to quit."
              }
              frame True {
                n129 = call "Stop Msg.vi"("error in (no error)"=w349, "Queue in"=w348) -> ("error out"=w347:errorcluster)  [unwired: 8 in, 1 out]
              }
            }
          }
        }
        n130 = property on="UI State" class="Enum (strict)"("Value"=w324) -> ()  [unwired: 2 in, 2 out]
      }
      frame "Exit" {
        w350 = UI_State."Idle" ("UI State")
        w361 = "Exit" ("Message")
        # "Popup an error dialog if 'Exit' was called as a result of an error."
        # "Stop the VI"
        # "Exit - Send Exit messages to the Acquisition and Logging loops, and fire the user event to stop the Event Handling Loop."
        n131 = Unbundle By Name(w354) -> ("Message Queues.Acquisition"=w353:refnum<queue>, "Message Queues.Logging"=w352:refnum<queue>)
        n132 = Variant To Data(type=errorcluster {"status"=FALSE, "code"=0, "source"=""} ("error constant"), Variant=w356) -> (data=w355:errorcluster)  [unwired: 1 in, 1 out]
        n133 = call <vilib>:"Simple Error Handler.vi"("error in (no error)"=w355) -> ()  [unwired: 4 in, 5 out]
        n134 = call-poly "Enqueue Message.vi"("Priority Message? (F)"=TRUE, "error in (no error)"=w358, "Message"=w361, "Message Queue"=w353) -> ("error out"=w362:errorcluster)  [unwired: 6 in, 1 out]
        n135 = call-poly "Enqueue Message.vi"("Priority Message? (F)"=TRUE, "error in (no error)"=w362, "Message"=w361, "Message Queue"=w352) -> ("error out"=w359:errorcluster)  [unwired: 6 in, 1 out]
        n136 = call "Fire User Event - Stop.vi"("error in (no error)"=w359, "User Event - Stop"=w365) -> ("error out"=w364:errorcluster)  [unwired: 9 in]
        n137 = property on="UI State" class="Enum (strict)"("Value"=w350) -> ()  [unwired: 2 in, 2 out]
      }
      frame Default {
        # "'Default' case only runs if there is a message that isn't defined in any of the other cases.  Output a programming error."
        n138 = xnode "Error Ring"("parameter 0"=w368) -> ("error out"=w367:errorcluster)
      }
    }
    n139 = call "Error Handler - Message Handling Loop.vi"("error in (no error)"=w27, "Message Queue"=w22) -> ("dup error in"=w28:errorcluster)  [unwired: 8 in, 1 out]
  }
  n140 = while {
    tunnel: w12 -> [w385]
    tunnel: [w382] -> w20
    shift-right: [w384] -> w15
    shift-left: w9 -> [w386]
    stop <- w383 stop-if-true
    # "UI Event Loop - Creates Messages for Handler"
    n141 = property on="UI State" class="Enum (strict)"() -> ("Value"=w378:T1)  [unwired: 2 in, 2 out]
    n142 = event shown="[0] \"Start\": Value Change" {
      selector: w386 -> [_ _ _ _ _ _ _ _]
      dyn-events: [_ _ _ _ _ _ _ _] -> w384
      timeout: 1000 -> [_ _ _ _ _ _ _ _]
      tunnel: [_ _ _ _ _ _ _ TRUE ("Discard?")] -> w383
      tunnel: w385 -> [w390 w392 w398 w402 w407 w410 w412 w416]
      tunnel: [w389 _ _ w401 w405 _ w415 _] -> w381
      tunnel: [w388 w391 w397 w400 w406 w410 w411 w416] -> w380
      tunnel: w378 -> [_ w393 _ _ _ _ _ _]
      event "Start": Value Change {
        (unwired) TRUE ("Time has Elapsed")
        n143 = event-data() -> ()  [unwired: 1 in, 1 out]
        n144 = call-poly "Enqueue Message.vi"("Message Array"=string[] ["Broadcast Settings", "Start"], "Message Queue"=w390) -> ("error out"=w389:errorcluster, "dup Message Queue"=w388:refnum<queue>)  [unwired: 8 in]
      }
      event Timeout {
        n145 = event-data() -> ()  [unwired: 1 in, 1 out]
        n146 = case shown="\"Acquiring and Logging\"" w393 {
          tunnel: w392 -> [w394 w395]
          tunnel: [w394 w396] -> w391
          frame "Idle", Default {
          }
          frame "Acquiring and Logging" {
            n147 = call "Has Time Elapsed Msg.vi"("UI Queue in"=w395) -> ("UI Queue out"=w396:refnum<queue>)  [unwired: 9 in, 1 out]
          }
        }
      }
      event "Settings": Value Change {
        n148 = event-data() -> ()  [unwired: 1 in, 1 out]
        n149 = call-poly "Enqueue Message.vi"("Message"="Launch Settings Dialog", "Message Queue"=w398) -> ("dup Message Queue"=w397:refnum<queue>)  [unwired: 8 in, 1 out]
      }
      event "Stop": Value Change {
        (unwired) FALSE ("Time has Elapsed")
        n150 = event-data() -> ()  [unwired: 1 in, 1 out]
        n151 = call-poly "Enqueue Message.vi"("Message"="Stop", "Message Queue"=w402) -> ("error out"=w401:errorcluster, "dup Message Queue"=w400:refnum<queue>)  [unwired: 8 in]
      }
      event Panel Close? {
        (unwired) FALSE ("Discard?")
        # "Send the 'Confirm Quit' message if the user closes the panel of the VI. Discard the event so the 'Confirm Quit' message has a chance to run."
        n152 = event-data() -> ()  [unwired: 1 in, 1 out]
        n153 = call-poly "Enqueue Message.vi"("Priority Message? (F)"=TRUE, "Message"="Confirm Quit", "Message Queue"=w407) -> ("error out"=w405:errorcluster, "dup Message Queue"=w406:refnum<queue>)  [unwired: 7 in]
        n154 = event-data("Discard?"=TRUE) -> ()  [unwired: 1 in, 1 out]
      }
      event Application Instance Close {
        (unwired) FALSE ("Time has Elapsed")
        n155 = event-data() -> ()  [unwired: 1 in, 1 out]
      }
      event "Exit": Value Change {
        w413 = TRUE  # Priority Message
        # "The UI Message Loop handles sending the Exit message to other loops."
        n156 = event-data() -> ()  [unwired: 1 in, 1 out]
        n157 = call-poly "Enqueue Message.vi"("Priority Message? (F)"=w413, "Message"="Exit", "Message Queue"=w412) -> ("error out"=w415:errorcluster, "dup Message Queue"=w411:refnum<queue>)  [unwired: 7 in]
      }
      event User Event {
        # "The Message Handling Loop processed an \"Exit\" message, which fired this event to stop the Event Handling Loop."
        n158 = event-data() -> ()  [unwired: 1 in, 1 out]
        n159 = local write "Status Bar"("Exit" ("Exit String")) -> ()
      }
    }
    n160 = call "Error Handler - Event Handling Loop.vi"("error in (no error)"=w381, "Message Queue"=w380) -> ("dup error in"=w382:errorcluster)  [unwired: 8 in, 1 out]
  }
  n161 = call "Logging Message Loop.vi"("error in (no error)"=w17, "Message Queues"=w2) -> ("error out"=w18:errorcluster)  [unwired: 9 in]
  n162 = call "Data Display Loop.vi"("Message Queues in"=w2, "WaveformChart in"=w5) -> ()  [unwired: 10 in]
  n163 = call "Acquisition Message Loop.vi"("error in (no error)"=w17, "Message Queues"=w2) -> ("error out"=w19:errorcluster)  [unwired: 9 in]
  n164 = call "ReleaseAllQueues.vi"("error in (no error)"=w21, "Message Queues"=w2) -> ("error out"=w10:errorcluster)  [unwired: 9 in]
  n165 = Unregister For Events(event registration refnum=w15, error in=w20) -> (error out=w16:errorcluster)
  n166 = Merge Errors(w16, w10, w19, w18) -> (w13:errorcluster)
  n167 = call "Destroy User Event - Stop.vi"("error in (no error)"=w13, "User Event - Stop"=w8) -> ("error out"=w11:errorcluster)  [unwired: 9 in]
  n168 = call "Close Executable.vi"("error in (no error)"=w11) -> ()  [unwired: 11 in]
